vi "Evaluate Part 2.vi"() -> ()   [LabVIEW 2021]
uses:
  Beam/Beam.lvclass/Beam.ctl
  Beam/Beam.lvclass
  Proto/Maze.lvclass
panel:
  out "Time [ms]":u32
  out "Max":i32
  in  "Input":string=".|...\\....\n|.-.\\.....\n.....|-...\n........|.\n..........\n.........\\\n..../.\\\\..\n.-.-/..|..\n.|....-|.\\\n..//.|...."
  # "Prallelll:\n1 630 354\n\nSingle Thread:\n 976 169"
  # "6883"
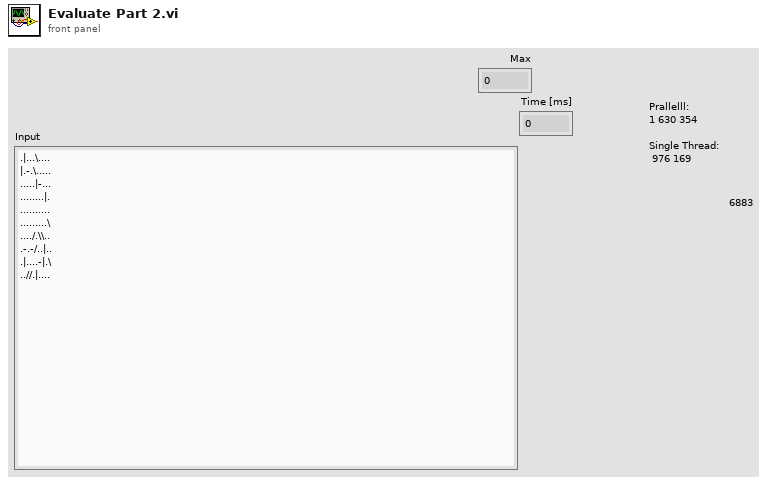
[diagram p1: front panel]
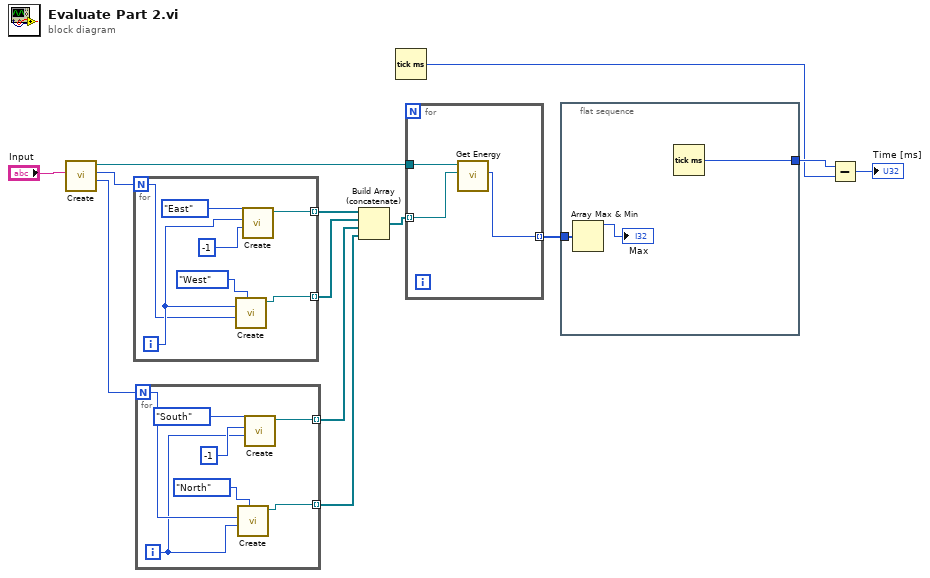
[diagram p0: block diagram]
diagram:
  n1 = call "Create.vi"("Input"="Input") -> ("Cols"=w6:i32, "Rows"=w9:i32, "Proto"=w12:refnum<class "Maze.lvclass">)  [unwired: 7 in, 1 out]
  n2 = for {
    N: w9 -> [w15]
    tunnel: [w18] -> w11 mode=indexing
    tunnel: [w14] -> w7 mode=indexing
    i -> [w16]
    n3 = call "Create.vi"("Direction"=enum16{"North", "East", "South", "West"}."West", "Col"=w15, "Row"=w16) -> ("Beam"=w14:refnum<class "Beam.lvclass">)  [unwired: 7 in, 1 out]
    n4 = call "Create.vi"("Direction"=enum16{"North", "East", "South", "West"}."East", "Col"=-1, "Row"=w16) -> ("Beam"=w18:refnum<class "Beam.lvclass">)  [unwired: 7 in, 1 out]
  }
  n5 = for {
    N: w6 -> [w23]
    tunnel: [w26] -> w5 mode=indexing
    tunnel: [w24] -> w4 mode=indexing
    i -> [w21]
    n6 = call "Create.vi"("Direction"=enum16{"North", "East", "South", "West"}."North", "Col"=w21, "Row"=w23) -> ("Beam"=w24:refnum<class "Beam.lvclass">)  [unwired: 7 in, 1 out]
    n7 = call "Create.vi"("Direction"=enum16{"North", "East", "South", "West"}."South", "Col"=w21, "Row"=-1 ("Col")) -> ("Beam"=w26:refnum<class "Beam.lvclass">)  [unwired: 7 in, 1 out]
  }
  n8 = Build Array (concatenate)(w11, w7, w5, w4) -> (w8:refnum<class "Beam.lvclass">[])
  n9 = Tick Count (ms)() -> (millisecond timer value=w2:u32)
  n10 = for {
    tunnel: [w29] -> w10 mode=indexing
    tunnel: w8 -> [w28] mode=indexing
    tunnel: w12 -> [w30]
    n11 = call "Get Energy.vi"("Beam"=w28, "Maze in"=w30) -> ("Numeric"=w29:i32)  [unwired: 8 in, 1 out]
  }
  n12 = flat-sequence {
    tunnel: w10 -> [w33]
    tunnel: [w31] -> w3
    frame #0 {
      n13 = Array Max & Min(array=w33) -> (max value=→"Max":i32)  [unwired: 3 out]
      n14 = Tick Count (ms)() -> (millisecond timer value=w31:u32)
    }
  }
  n15 = Subtract(x=w3, y=w2) -> (x-y=→"Time [ms]":u32)
